vi "HEWH SUo Start Index.vi"(8 "error in (no error)":errorcluster, 9 "Test Data-Start to End DBL":dbl[][](array[numeric]), 10 "Draw Index in":i32[](array[numeric]), 11 "Heating Index":i32[][](array[numeric])) -> (0 "error out":errorcluster, 3 "SUo Start Index":i32, 5 "Take Sample at 5 Min":bool)   [LabVIEW 2019]
panel:
  out "Software Timestamp":dbl
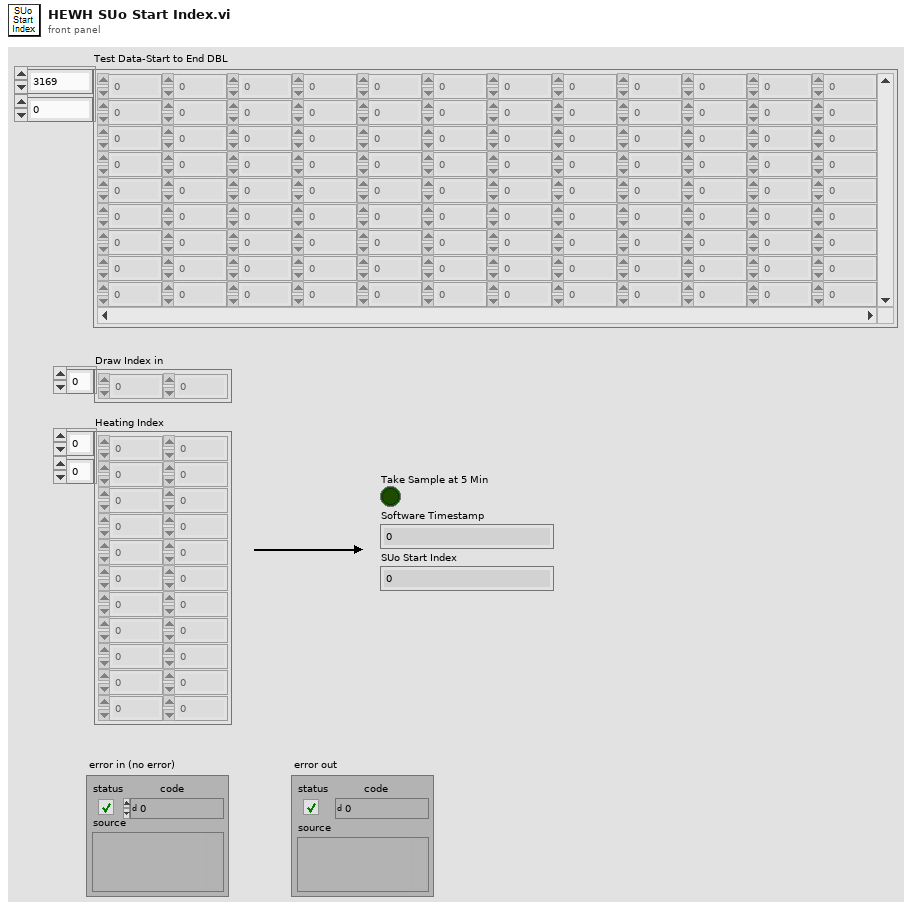
[diagram p1: front panel]
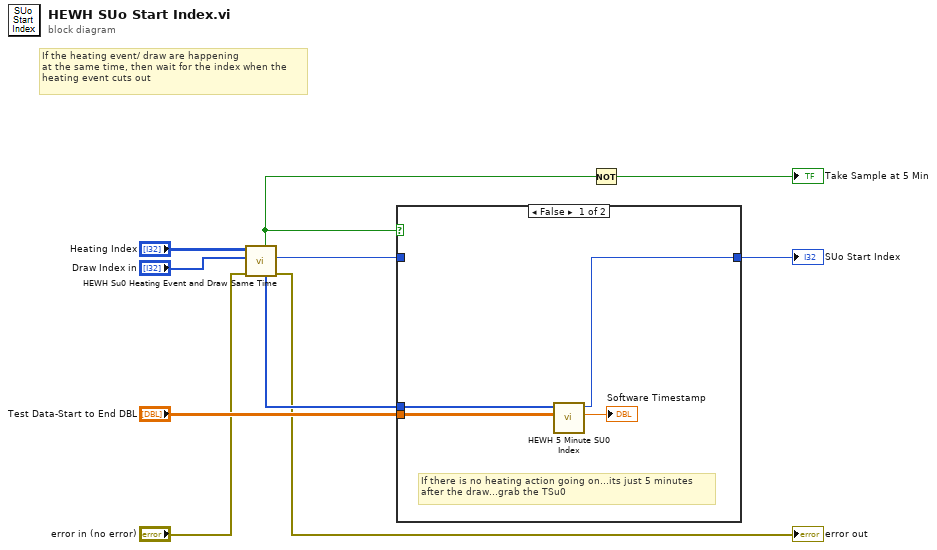
[diagram p0: block diagram]
diagram:
  # "If the heating event/ draw are happening\nat the same time, then wait for the index when the\nheating event cuts out"
  n1 = call "HEWH Su0 Heating Event and Draw Same Time.vi"("error in (no error)"="error in (no error)", "Draw Index in"="Draw Index in", "Heating Index in"="Heating Index") -> ("error out"=→"error out":errorcluster, "SUo Start Index"=w1:i32, "Draw Index out"=w8:i32[], "Heating Event Happening due to Draw?"=w4:bool)  [unwired: 5 in]
  n2 = case shown="False" w4 {
    tunnel: [w13 w15] -> w9
    tunnel: w8 -> [w14 _]
    tunnel: "Test Data-Start to End DBL" -> [w12 _]
    tunnel: w1 -> [_ w15]
    frame False {
      # "If there is no heating action going on...its just 5 minutes\nafter the draw...grab the TSu0"
      n3 = call "HEWH 5 Minute SU0 Index.vi"("Test Data-Start to End DBL"=w12, "Draw Index in"=w14) -> ("TSUo Software Timestamp"=→"Software Timestamp":dbl, "TSUo Index"=w13:i32)  [unwired: 7 in, 1 out]
    }
    frame True {
    }
  }
  "SUo Start Index" <- w9
  n4 = Not(x=w4) -> (.not. x?=→"Take Sample at 5 Min":bool)
